vi "mapping final edition.vi"() -> ()   [LabVIEW 2018]
uses:
  <vilib>/DAQmx/read.llb/DAQmx Read (Analog 2D DBL NChan NSamp).vi
  <vilib>/DAQmx/create/channels.llb/DAQmx Create Channel (AI-Voltage-Basic).vi
  <vilib>/DAQmx/configure/timing.llb/DAQmx Timing (Sample Clock).vi
  <vilib>/DAQmx/miscellaneous.llb/DAQmx Fill In Error Info.vi
  <vilib>/Utility/file.llb/Write Delimited Spreadsheet (DBL).vi
panel:
  in  "Path":path
  out "array size":i32
  out "AI2":dbl=981483.9601007936 format="%.9f"
  out "AI2":sgl=0.9249536 format="%.3f"
  in  "Start Scan":bool
  in  "x start":sgl format="%.4f"
  out "sec":sgl=9.0 format="%.3f"
  out "min":sgl=2.0 format="%.3f"
  out "hr":sgl format="%.3f"
  out "scaled data":sgl[][](array[numeric])=[[0.08995186, -0.065358415, 0.046570934, -0.028403355, 0.011250414, 0.0097677205, -0.036845274, 0.08059889, -0.15414652, 3.8100245, 5.301704, 4.7763147, 5.1208405, 4.852381, 5.0800614, 4.8759155, 5.0671434, 4.879784, 5.073785, 4.854985, 5.1510253, 4.4088683, 0.19852792, -0.05369336, 0.042853996, -0.04278115, 0.046836343, -0.05056593, 0.057532918, -0.06434656, 0.07648512, -0.09306003, 0.12637737, -0.20857362, 0.7113754, 4.8934565, 4.9863224, 4.9517126, 5.008813, 4.9254646, 5.0359926, 4.8951178, 5.072542, 4.84753, 5.14237, 4.7289605, 5.41226, 3.039946, -0.3712578, 0.1811235, -0.102439806, 0.057444878, -0.02437124, -0.0019917544, 0.0284711, -0.055142883, 0.08947336, -0.13621256, 0.21908402, -0.42042786, 2.049878, 5.3894496, 4.758692, 5.1075525, 4.8870254, 5.0276275, 4.9465346, 4.976245, 4.9966516, 4.9206614, 5.0678873, 4.810496, 5.2940927, 1.5762044, -0.37725365, 0.20376839, -0.13209367, 0.091401376, -0.061783113, 0.038824435, -0.016206224, -0.005852878, 0.033383638, -0.07024288, 0.13338381, -0.2740278, 3.4729016, 5.3619275, 4.748465, 5.1354837, 4.846731, 5.0798483, 4.8825455, 5.0552025, 4.899335, 5.0453405, 4.898891, 5.074322, 4.648711, 0.41327354, -0.12288489, 0.0801944, -0.06521296, 0.05908707, -0.05554355, 0.055086855, -0.055220723, 0.0584478, -0.06400715, 0.07833402, -0.11937849, 0.401842, 4.63731, 5.0785136, 4.8963833, 5.0473413, 4.897698, 5.056591, 4.88092, 5.0812073, 4.844774, 5.1375537, 4.7452354, 5.367524, 3.4397311, -0.28283846, 0.13752055, -0.072798684, 0.035415, -0.007555047, -0.01475798, 0.03739533, -0.060410146, 0.09001565, -0.13058291, 0.20192842, -0.3742972, 1.560797, 5.291227, 4.811963, 5.0674405, 4.921157, 4.9965672, 4.9762244, 4.9467287, 5.0273952, 4.8875346, 5.1069274, 4.759733, 5.3872814, 2.030668, -0.41930884, 0.21865785, -0.13621894, 0.08957672, -0.05563924, 0.028855167, -0.002696095, -0.023640106, 0.056296494, -0.10112171, 0.17909977, -0.3670662, 3.0687323, 5.4088187, 4.730429, 5.1410356, 4.8483744, 5.071446, 4.8960123, 5.034976, 4.926784, 5.007408, 4.9539905, 4.9831657, 4.9024124, 0.72391576, -0.2121617, 0.12789325, -0.0943156, 0.07678369, -0.06477019, 0.057225406, -0.050254583, 0.045999296, -0.041641697, 0.040820073, -0.050278828, 0.18801892, 4.394757, 5.155556, 4.8520226, 5.076152, 4.877726, 5.069264, 4.873699, 5.082649, 4.849418, 5.124974, 4.770708, 5.312019, 3.7631257, -0.1722489, 0.08832625, -0.04115682, 0.012989575, 0.009221593, -0.026924489, 0.045944422, -0.065192536, 0.090805486, -0.1260621, 0.18888147, -0.34058186, 1.3266691, 5.213644, 4.8505197, 5.040275, 4.943368, 4.9778323, 4.993703, 4.9309473, 5.0431857, 4.8718643, 5.123718, 4.7399697, 5.416989, 2.3209786, -0.4270834, 0.2178795, -0.13206305, 0.08381564, -0.048057344, 0.020409431, 0.007566642, -0.03510993, 0.07040888, -0.11812037, 0.20245795, -0.40821925, 2.750202, 5.425666, 4.7273817, 5.137802, 4.8552256, 5.06122, 4.9094777, 5.01756, 4.9486656, 4.97851, 4.9933968, 4.920391, 5.0557537, 0.97315127, -0.27107772, 0.15618311], [1.6148105, 0.6412399, 0.12259479, 0.10007006, 0.05627404, 0.11792919, 0.07558805, 0.096587755, 0.13539684, 0.18154798, 0.14659481, 0.14001909, 0.15269747, 0.32605436, 1.2285366, 1.8071078, 1.723693, 1.8642299, 1.8861247, 1.7781298, 1.7665774, 1.6843293, 1.6618632, 1.8358308, 1.7840756, 1.886492, 1.4087651, 0.34988096, 0.17499523, 0.13713227, 0.14069235, 0.14307298, 0.15526807, 0.16397195, 0.16420785, 0.15337072, 0.103284605, 0.13004267, 0.0764462, 0.37955138, 1.4378004, 1.7283472, 1.6601341, 1.9107368, 1.981662, 1.9060649, 1.7642057, 1.8262956, 1.8092386, 1.8622408, 1.7110121, 1.835776, 1.0515572, 0.23552063, 0.18500735, 0.110096216, 0.11694353, 0.05356826, 0.11541723, 0.099398084, 0.09107675, 0.13544913, 0.09703531, 0.11242456, 0.118112795, 0.69184244, 1.4759477, 1.6194212, 1.8840069, 1.9284915, 1.8578812, 1.8474318, 1.8391486, 1.8397951, 1.8988006, 1.9207095, 1.7646545, 1.7554979, 0.7396219, 0.22156206, 0.15757602, 0.12271975, 0.1853172, 0.1761696, 0.16238572, 0.17065349, 0.12731779, 0.09591067, 0.09957277, 0.15292062, 0.100816004, 0.977814, 1.6875081, 1.8349446, 1.8618723, 1.7646685, 1.7791893, 1.7086927, 1.8239698, 1.9180751, 1.8788452, 1.7875822, 1.9220088, 1.4754479, 0.44321483, 0.13592602, 0.084151655, 0.08818737, 0.1107886, 0.15709913, 0.18759453, 0.15712845, 0.18021806, 0.17567357, 0.17235321, 0.12586543, 0.40349913, 1.447578, 1.674117, 1.8619998, 1.9170333, 1.8629906, 1.8370001, 1.8740305, 1.9876027, 1.8765373, 1.7414004, 1.6534603, 1.8096567, 1.1517842, 0.287448, 0.20285116, 0.066186704, 0.08846406, 0.11164929, 0.13587119, 0.15773286, 0.14254764, 0.10292374, 0.12034805, 0.15531144, 0.12162699, 0.6911105, 1.593376, 1.892207, 1.8803179, 1.9277658, 1.9091481, 1.860953, 1.9320847, 1.8267941, 1.8986298, 1.8120731, 1.6568379, 1.6279173, 0.781555, 0.19091108, 0.12488488, 0.08304486, 0.105652474, 0.11557407, 0.1490494, 0.09324315, 0.07362821, 0.0935173, 0.14308317, 0.15568249, 0.11385268, 0.87998796, 1.6663209, 1.8585353, 2.016943, 1.9768472, 1.8131237, 1.851382, 1.9297907, 1.8807145, 1.8564926, 1.8491366, 1.9471296, 1.5421423, 0.546228, 0.2057074, 0.20138735, 0.111848205, 0.08376657, 0.14174303, 0.16643672, 0.078453206, 0.116940975, 0.12531969, 0.098607525, -0.00568714, 0.2587199, 1.2634019, 1.6675119, 1.648064, 1.7753998, 1.9649504, 1.7998588, 1.7356408, 1.7368636, 1.6777064, 1.8816746, 1.8367412, 1.8527502, 1.2181253, 0.3530853, 0.21028247, 0.09459221, 0.1144762, 0.10214721, 0.092193745, 0.062590905, 0.115664594, 0.09098494, 0.115862235, 0.09943251, 0.069180645, 0.4846417, 1.4973682, 1.8450817, 1.8296045, 1.8144448, 1.7862815, 1.799637, 1.9097167, 1.8960272, 1.7957402, 1.7565843, 1.7647425, 1.8072952, 0.8449825, 0.1833395, 0.18335354, 0.031213127, 0.09104742, 0.12451765, 0.15377748, 0.09247936, 0.13039716, 0.17976157, 0.1752885, 0.16731273, 0.18515654, 0.9803604, 1.7406315, 1.85674, 1.8916562, 1.7167296, 1.7266883, 1.7743402, 1.8966228, 1.7989038, 1.7762464, 1.8464664], [-1.4767952, -0.52093244, -0.065139994, -0.04381245, -0.015159501, -0.023012077, 0.030354373, 0.004124446, -0.037436225, -0.03062673, -0.049429834, -0.038981438, -0.05951384, -0.12666832, -0.96224815, -1.4578644, -1.417214, -1.6564966, -1.5031904, -1.4855494, -1.5529104, -1.5899595, -1.6205446, -1.4851049, -1.3304464, -1.4843547, -1.1244048, -0.3124867, -0.09511276, -0.0067108776, 0.008348133, -0.06884276, -0.028149867, 0.0060778856, 0.014657993, 0.0035960134, 0.029784627, -0.001404034, -0.010573929, -0.23944686, -1.1427158, -1.592673, -1.6138891, -1.5006585, -1.5761764, -1.6237564, -1.6302592, -1.4553976, -1.4390112, -1.5583963, -1.6095014, -1.6356761, -0.8941107, -0.14872715, -0.04852324, -0.016287742, -0.0072004925, 0.05171574, 0.024102116, -0.03878735, -0.029223012, 0.0013796147, 0.0007109344, -0.09832217, -0.026550805, -0.57925135, -1.3799185, -1.4696552, -1.5014336, -1.6099834, -1.6062907, -1.5134172, -1.4725603, -1.4464005, -1.471114, -1.6949456, -1.6740988, -1.443826, -0.5317577, -0.096025616, -0.095088966, -0.01003298, -0.030934773, -0.03786698, -0.066740304, -0.028596912, -0.0075047743, -0.045842268, -0.028847354, 0.017677061, -0.06430727, -0.91461426, -1.5800095, -1.6365865, -1.669164, -1.6613489, -1.5563904, -1.6387641, -1.621947, -1.6419398, -1.5808084, -1.4260033, -1.746947, -1.4109493, -0.31155756, -0.03549656, -0.0893977, -0.0493835, -0.02766151, -0.055632003, -0.020448817, -0.03490928, -0.0065092742, -0.0044493936, -0.008321209, 0.03713632, -0.22255462, -1.256689, -1.6435188, -1.58099, -1.6661974, -1.6825287, -1.7567831, -1.6967863, -1.6964307, -1.5608094, -1.5687697, -1.5021436, -1.7775272, -1.1238, -0.18753046, -0.06339442, 0.033160567, -0.037432462, -0.0655407, 0.012275046, 0.019751964, -0.074713096, -0.059357315, 0.017791009, -0.004530791, 0.051316284, -0.45699736, -1.4750546, -1.6812614, -1.6400126, -1.5128337, -1.5886396, -1.4835271, -1.558737, -1.5912981, -1.5443467, -1.5120009, -1.5561036, -1.5510322, -0.6751001, -0.13700025, -0.070947714, 0.029946156, -0.06867997, -0.0646341, -0.023216186, 0.022019707, -0.00063267536, -0.049820524, 0.08989921, 0.031814445, -0.01631529, -0.76614785, -1.5538985, -1.7605923, -1.8131211, -1.615681, -1.6916823, -1.5543268, -1.4462615, -1.5637659, -1.6425695, -1.5686895, -1.6034069, -1.3314981, -0.39967144, -0.1255188, -0.042046838, -0.05730996, -0.059426185, -0.054224525, -0.0747444, 0.004988471, -0.03528243, -0.036589727, -0.0626456, -0.030736923, -0.1435518, -1.0285323, -1.4818504, -1.4843473, -1.4634567, -1.4524511, -1.5054933, -1.5445257, -1.5867013, -1.5180717, -1.6029373, -1.6105895, -1.7413071, -1.0346706, -0.19276091, -0.12739836, -0.015712976, -0.051736392, -0.0066845864, 0.0036811642, -0.018952433, -0.008254843, 0.023332015, 0.015603406, 0.005991487, 0.005503129, -0.3153793, -1.1979393, -1.4788326, -1.5864795, -1.5806519, -1.5993572, -1.5863644, -1.4998145, -1.6164098, -1.6253455, -1.5748917, -1.7109123, -1.6193199, -0.67024153, -0.121727124, -0.092952706, -0.02475514, -0.026037404, 0.034906138, -0.02021716, -0.03959001, -0.008375058, -0.047745623, -0.024242997, -0.06765317, -0.029479712, -0.7310273, -1.4417034, -1.4696852, -1.4992273, -1.62077, -1.7575307, -1.5015112, -1.5808134, -1.6111705, -1.6930485, -1.6120521]] format="%0.6f"
  in  "Physical Channel":tag="Dev2/ai0:2"
  in  "AI Rate":dbl=5120.0 format="%.2f"
  out "X Position":sgl=5.7001514 format="%.4f"
  out "AI0":dbl=1080521.7918445107 format="%.9f"
  out "AI1":dbl=981483.9601007936 format="%.9f"
  out "Y Position":sgl=0.6143307 format="%.4f"
  out "necessary time (s)":dbl=129.0
  in  "Time/Step(ms)":u32=1000 min=1 step=1
  out "For_Home":dbl=0.5
  in  "Motor HWSerialNum A":u32=83827753
  out "error":errorcluster
  in  "Channel A":i32
  in  "Channel B":i32
  in  "Both Channels":i32=10
  in  "MG17Motor A":refnum<k7>(container)
  in  "MG17Motor B":refnum<k7>(container)
  in  "Motor HWSerialNum B":u32=83827752
  in  "Error":errorcluster
  in  "Z Scale.Range:Minimum":dbl=0.5
  in  "Z Scale.Range:Maximum":dbl=10.0
  in  "Pixels(Y)":i32=10
  out "x .and. y?":bool=TRUE
  out "AI1 Reading":sgl=1916.9768 caption="AI1" format="%.3f"
  out "AI0 Reading":sgl=1773.1146 caption="AI0" format="%.3f"
  out "AI2":dbl[][](graph)
  out "Outphase Array":dbl[][](array[numeric])=[[2562.4082924284185, 1817.6676888834427, 2051.3325671838757, 1598.5840726397216, 2356.139803338449, 2083.283068035537, 2141.9285945761453, 2438.1745524803077, 1984.8193530672331, 2518.2976810936884], [2013.6293646842878, 2905.788176064875, 2403.5143450391743, 2075.1285214946324, 1794.2852932607746, 2154.2324476248573, 2573.051600709472, 2289.9591852377134, 1840.6423205131646, 3056.691954941658], [1462.7563247041599, 2489.6853377240786, 3113.7141928608366, 2094.263243597831, 1980.880488063484, 2798.2521113290636, 3180.218346584931, 1955.014012814602, 1954.9062009375507, 2330.0172899718864], [2654.506466159619, 1706.9104786367188, 2763.849371509579, 2665.4676788285865, 3132.939147321313, 1990.492248608471, 3191.66238810395, 2902.203788288949, 2369.1083072617203, 2413.0030199350244], [2875.5255335084453, 1413.9419064107196, 2133.996309941279, 1582.8516778375904, 2285.5732989580556, 2032.7550230687993, 1403.1269673599186, 2348.5457130522527, 2793.543648369003, 2638.42704917987], [2508.860871301475, 2017.0923640774959, 2103.4938570285726, 2506.6668144539026, 2520.3189193813937, 1623.1935507015144, 2117.008235660878, 1990.9220243912062, 2369.004550581991, 1817.1745751417288], [2127.008781202753, 1894.076946993543, 2350.908791062092, 1608.5249433544752, 2367.4088747592477, 2261.8591956234536, 2856.9839458223373, 1944.1817298861051, 2606.7766866868633, 1847.702813397054], [1332.3239444506978, 3089.345384527674, 3117.6849510516045, 1823.2018060552239, 2907.347843840017, 2513.6901896156223, 1883.004697534108, 2598.892861462688, 2158.04090585742, 2821.9623698891833], [2783.620807424688, 3090.3816841375274, 2126.982362670075, 1802.3502961996567, 2121.8058461401215, 1389.8670829981122, 2695.1174997292997, 1862.877057878669, 1123.7561431306951, 3173.8482288755017], [3289.294215227313, 3427.646935048104, 1868.9893279501098, 1265.6961355991489, 3028.863630242435, 2568.628200265615, 2625.960251038055, 2112.3260575013605, 2293.5876318191563, 1916.9768566871817], [0.0, 0.0, 0.0, 0.0, 0.0, 0.0, 0.0, 0.0, 0.0, 0.0], [0.0, 0.0, 0.0, 0.0, 0.0, 0.0, 0.0, 0.0, 0.0, 0.0], [0.0, 0.0, 0.0, 0.0, 0.0, 0.0, 0.0, 0.0, 0.0, 0.0], [0.0, 0.0, 0.0, 0.0, 0.0, 0.0, 0.0, 0.0, 0.0, 0.0], [0.0, 0.0, 0.0, 0.0, 0.0, 0.0, 0.0, 0.0, 0.0, 0.0], [0.0, 0.0, 0.0, 0.0, 0.0, 0.0, 0.0, 0.0, 0.0, 0.0], [0.0, 0.0, 0.0, 0.0, 0.0, 0.0, 0.0, 0.0, 0.0, 0.0], [0.0, 0.0, 0.0, 0.0, 0.0, 0.0, 0.0, 0.0, 0.0, 0.0], [0.0, 0.0, 0.0, 0.0, 0.0, 0.0, 0.0, 0.0, 0.0, 0.0], [0.0, 0.0, 0.0, 0.0, 0.0, 0.0, 0.0, 0.0, 0.0, 0.0]]
  out "Inphase Array":dbl[][](array[numeric])=[[2044.6463625125714, 2048.007662191087, 1857.2525864253337, 2367.536167113699, 1677.5847421288915, 3518.7700021734063, 3017.990323192611, 1790.35736608951, 973.9359143332003, 1961.5367899300145], [1674.8440274838545, 2393.3161888851737, 3047.069407355723, 2831.9502902122717, 2575.6596526949597, 2640.3955094250277, 2707.38612778617, 2752.6705551580535, 2601.6534846507584, 2428.802308846195], [2310.539174707911, 2019.4980579908167, 1695.4316967259595, 3165.8313269644823, 2974.8805843760015, 2521.9709412910042, 1332.5610352925755, 1952.563600677248, 2877.336113219085, 1895.061160929894], [3252.8926277691635, 2822.4440682237696, 2634.978174426852, 2361.470345238801, 2106.861238475591, 2470.3862405323457, 2504.170845974706, 2514.8891074351964, 1680.5844638621936, 2858.877309939785], [2768.0539491905397, 2186.0164703118107, 2539.6366460966865, 2640.577817303329, 3117.019873675447, 2573.625813695958, 1976.3462073162439, 2035.7740034242272, 1545.9525168596529, 2242.6229061407557], [1874.3233177350737, 2505.741725715464, 2783.8180046186562, 1842.768823260741, 2555.264741602122, 2882.3282081275916, 2818.5003810212797, 3251.099795547098, 2569.4618761698066, 1322.899149168236], [1540.9844582418293, 2057.077993816449, 2495.5409296646358, 1977.5648561441858, 2223.188598020489, 2486.5520399883585, 1586.5726572114816, 2615.9088005342264, 1254.4943744059751, 2253.562060012856], [2955.7185549552687, 2750.74135698765, 1818.3861337580702, 2572.2228754086773, 2137.553351193629, 1375.2105871652152, 3355.1487666885364, 2141.5017884888475, 2734.5506302466356, 1843.7281765812454], [1858.2546438169445, 1583.66230481497, 2611.782079607164, 3046.8759742374796, 1529.7603908309666, 1274.6513951532384, 2276.057074441497, 2421.2195908700114, 2331.4669215367194, 3086.2871139714543], [2460.676783449499, 1393.87787290715, 2469.907081701711, 2303.007218218374, 1704.4213840891673, 1594.5417502298358, 2147.1556828119224, 2407.7757693353487, 1540.0436035810508, 1773.1145717006036], [0.0, 0.0, 0.0, 0.0, 0.0, 0.0, 0.0, 0.0, 0.0, 0.0], [0.0, 0.0, 0.0, 0.0, 0.0, 0.0, 0.0, 0.0, 0.0, 0.0], [0.0, 0.0, 0.0, 0.0, 0.0, 0.0, 0.0, 0.0, 0.0, 0.0], [0.0, 0.0, 0.0, 0.0, 0.0, 0.0, 0.0, 0.0, 0.0, 0.0], [0.0, 0.0, 0.0, 0.0, 0.0, 0.0, 0.0, 0.0, 0.0, 0.0], [0.0, 0.0, 0.0, 0.0, 0.0, 0.0, 0.0, 0.0, 0.0, 0.0], [0.0, 0.0, 0.0, 0.0, 0.0, 0.0, 0.0, 0.0, 0.0, 0.0], [0.0, 0.0, 0.0, 0.0, 0.0, 0.0, 0.0, 0.0, 0.0, 0.0], [0.0, 0.0, 0.0, 0.0, 0.0, 0.0, 0.0, 0.0, 0.0, 0.0], [0.0, 0.0, 0.0, 0.0, 0.0, 0.0, 0.0, 0.0, 0.0, 0.0]]
  out "Ratio Array":dbl[][](array[numeric])=[[0.7979393325233274, 1.1267228188718796, 0.9053883393344746, 1.4810207405633764, 0.7120056032973499, 1.689050353340357, 1.4090060382194136, 0.7343023756310696, 0.4906924717496996, 0.7789137895239316], [0.831753875294945, 0.8236375275386695, 1.267755864925391, 1.364710793032005, 1.4354794426332196, 1.2256780888878487, 1.0522082522712166, 1.2020609681182188, 1.4134486943261342, 0.7945852394185899], [1.5795790014274689, 0.8111459016089644, 0.544504598595872, 1.5116682855617305, 1.5017971060355364, 0.9012665195821701, 0.4190155800854185, 0.9987466012410693, 1.4718537962788942, 0.8133249350062803], [1.2254227553173958, 1.65353959891207, 0.9533725685592123, 0.8859497205670919, 0.6724871245191512, 1.241093122698349, 0.7845976614908642, 0.8665446298372791, 0.7093742648704224, 1.184779830908279], [0.9626254112281246, 1.546044049193645, 1.1900848348545503, 1.668240842951722, 1.3637803150292447, 1.266077704636843, 1.4085298431936473, 0.8668232396372918, 0.5534019551698252, 0.8499848069848487], [0.7470814102030161, 1.2422543312048324, 1.3234257829262785, 0.7351470935965628, 1.0138656350003934, 1.775714428437633, 1.3313601400050354, 1.632961891885864, 1.084616690811577, 0.7279978309541656], [0.7244842954388057, 1.0860583024790185, 1.0615217992090633, 1.2294275350310089, 0.9390809596616785, 1.09933989029895, 0.5553313169755358, 1.3455063178108728, 0.4812435145721672, 1.2196561285034893], [2.218468389212864, 0.8903961890321975, 0.5832488408248958, 1.4108272967182252, 0.7352244953154125, 0.5470883376346007, 1.7818058399335261, 0.8240054140914392, 1.2671449474495295, 0.6533496676830767], [0.6675674498697756, 0.5124487738662427, 1.2279284141916924, 1.690501552701473, 0.7209709567036149, 0.9171030890260818, 0.8445112595907625, 1.299720548186443, 2.07470894445252, 0.9724116880865881], [0.7480865567020885, 0.4066573656272997, 1.321520163205363, 1.8195577543801127, 0.5627263529037597, 0.6207756148067473, 0.8176649596897521, 1.1398693685497927, 0.6714561860274626, 0.9249535619145693], [0.0, 0.0, 0.0, 0.0, 0.0, 0.0, 0.0, 0.0, 0.0, 0.0], [0.0, 0.0, 0.0, 0.0, 0.0, 0.0, 0.0, 0.0, 0.0, 0.0], [0.0, 0.0, 0.0, 0.0, 0.0, 0.0, 0.0, 0.0, 0.0, 0.0], [0.0, 0.0, 0.0, 0.0, 0.0, 0.0, 0.0, 0.0, 0.0, 0.0], [0.0, 0.0, 0.0, 0.0, 0.0, 0.0, 0.0, 0.0, 0.0, 0.0], [0.0, 0.0, 0.0, 0.0, 0.0, 0.0, 0.0, 0.0, 0.0, 0.0], [0.0, 0.0, 0.0, 0.0, 0.0, 0.0, 0.0, 0.0, 0.0, 0.0], [0.0, 0.0, 0.0, 0.0, 0.0, 0.0, 0.0, 0.0, 0.0, 0.0], [0.0, 0.0, 0.0, 0.0, 0.0, 0.0, 0.0, 0.0, 0.0, 0.0], [0.0, 0.0, 0.0, 0.0, 0.0, 0.0, 0.0, 0.0, 0.0, 0.0]]
  in  "st(mm/step)":dbl=2.0 format="%_1f"
  in  "Pixels(X)":i32=10
  # "Necessary Time"
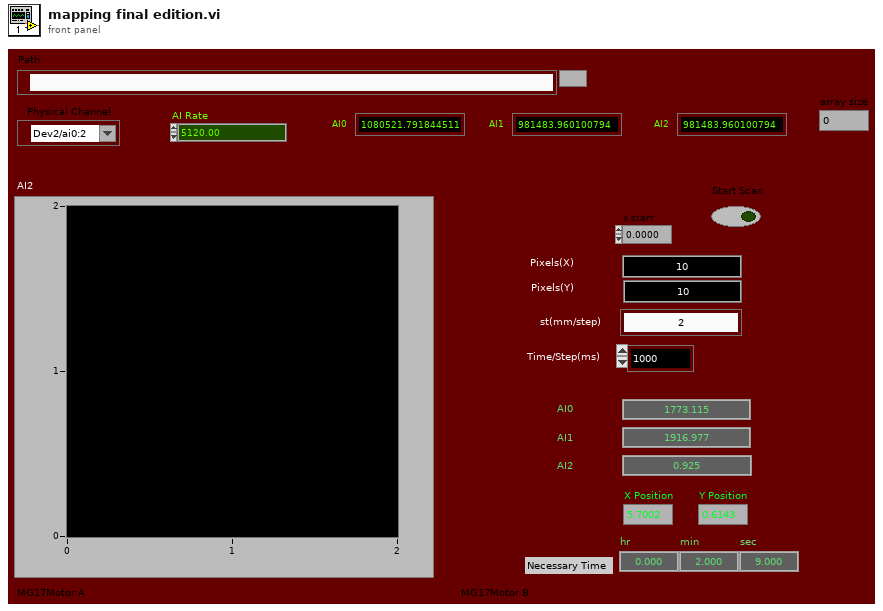
[diagram p1: front panel]
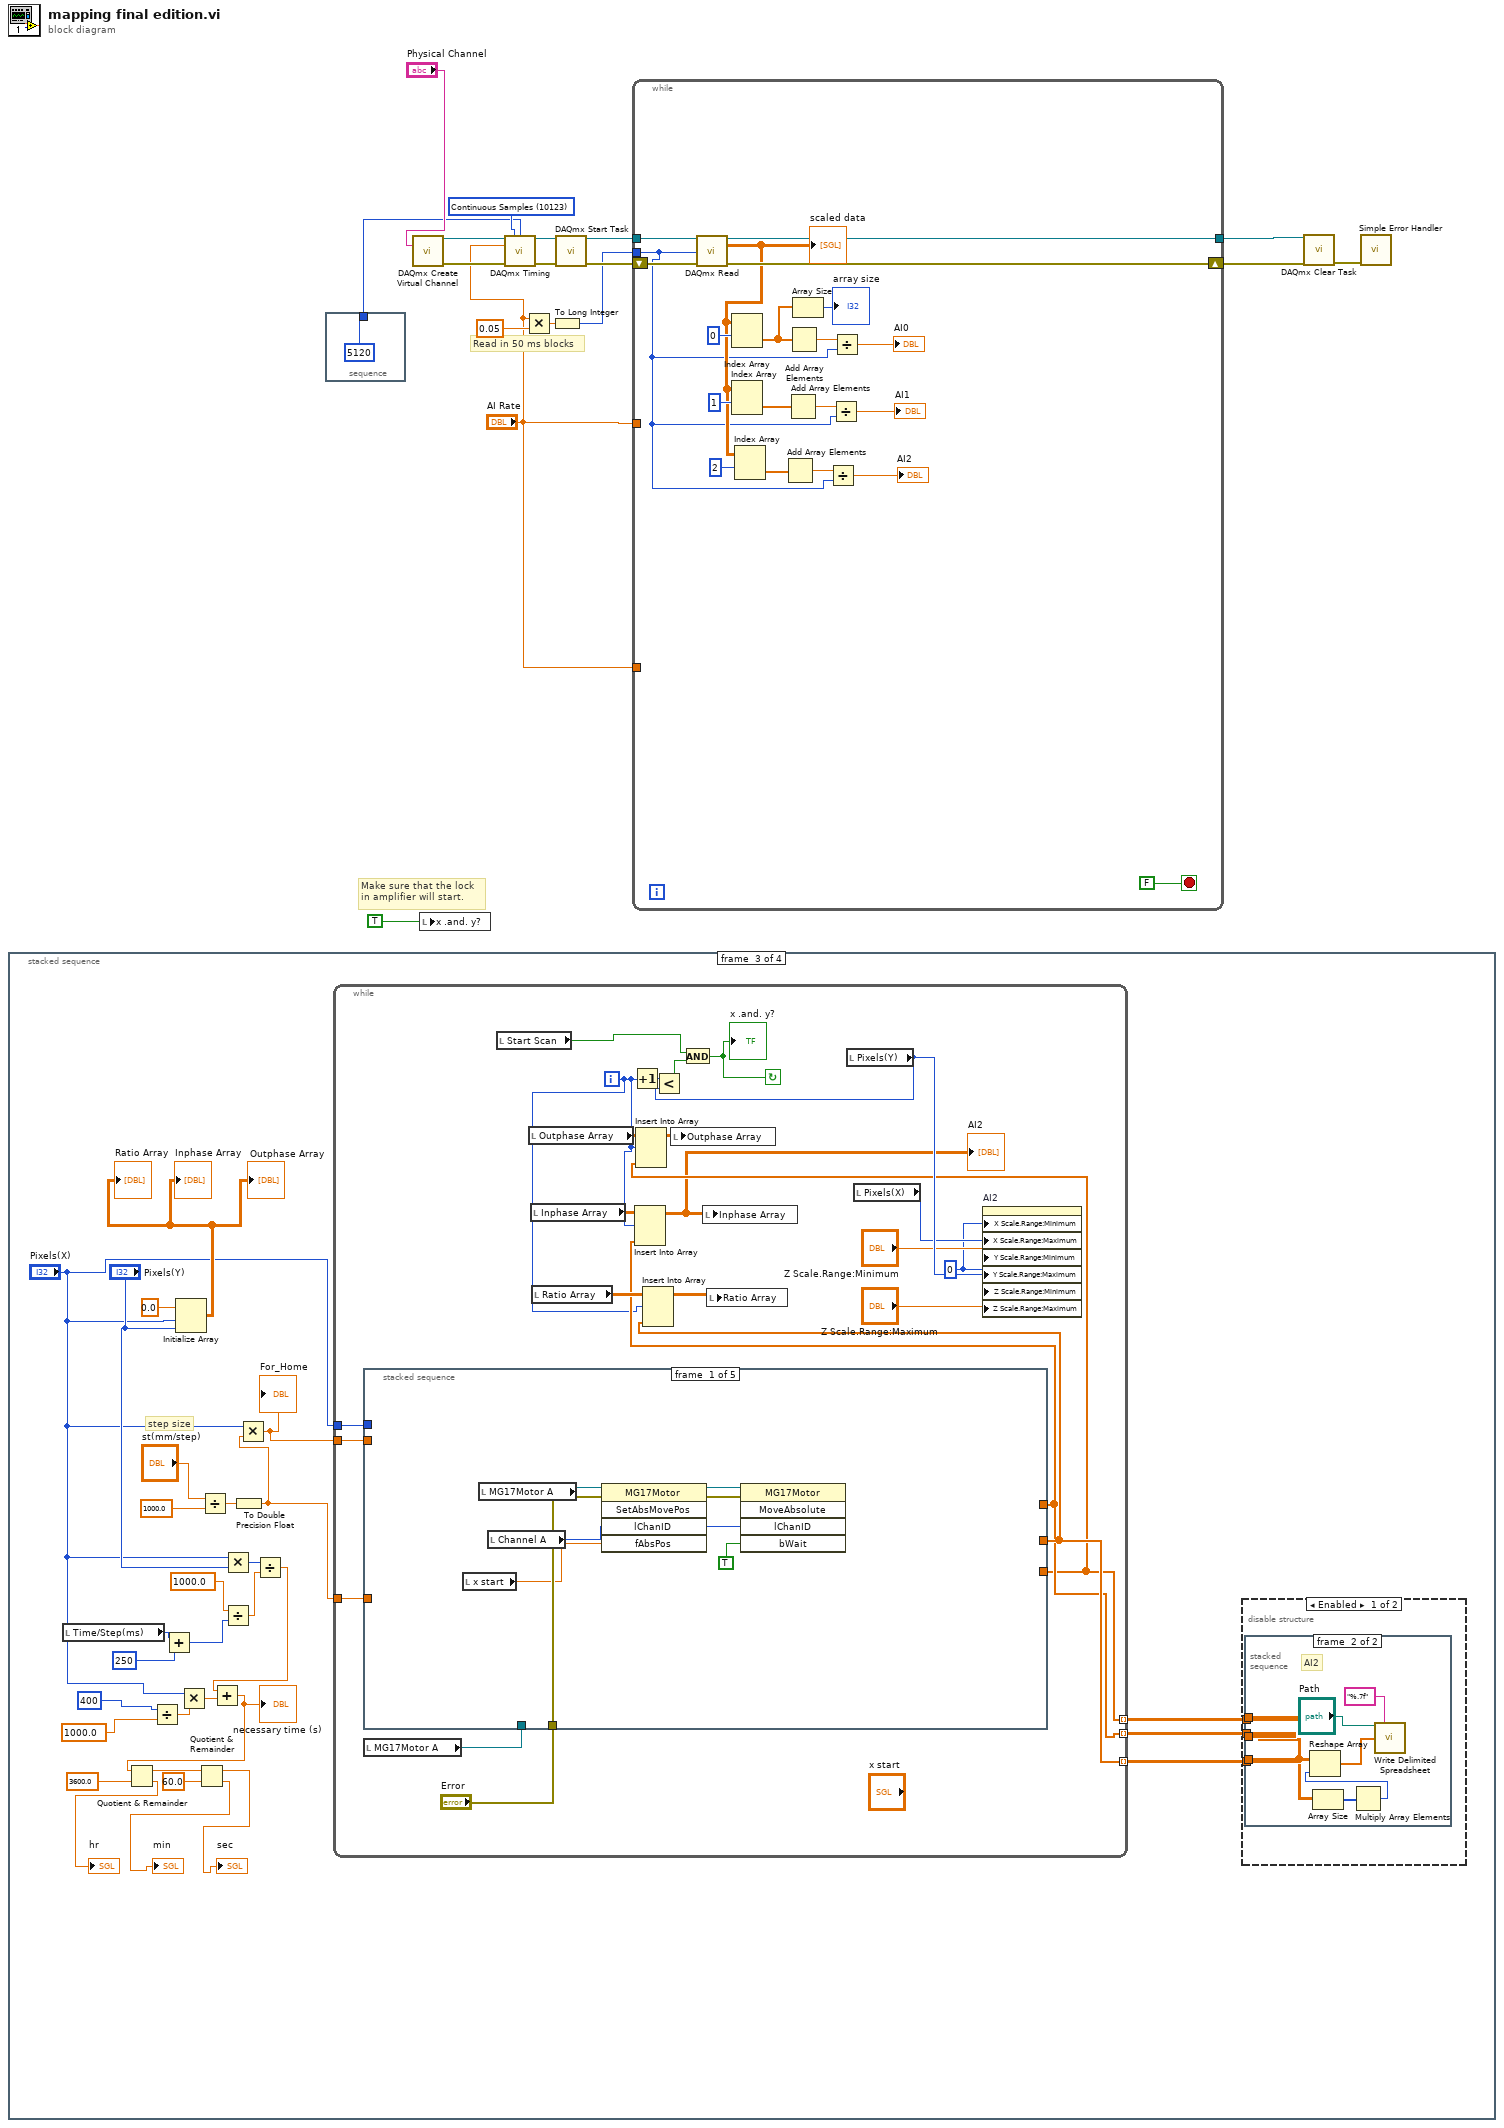
[diagram p0: block diagram]
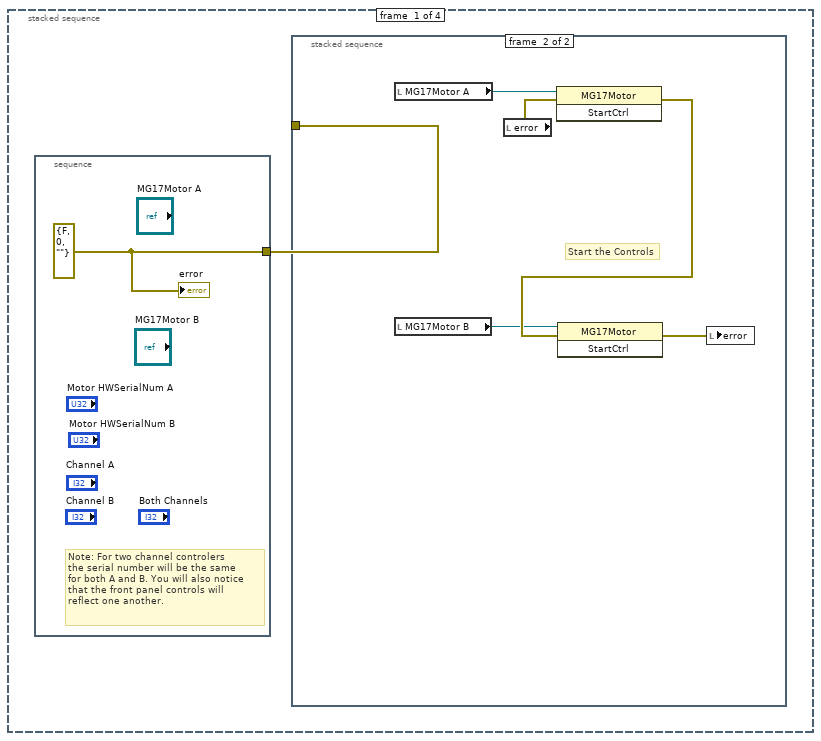
[diagram p2: hidden frame]
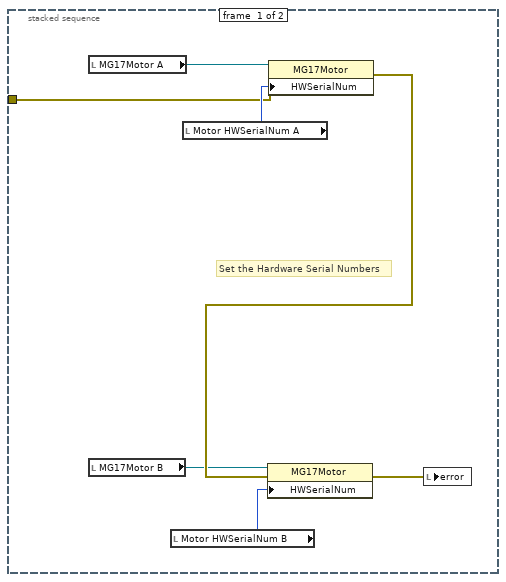
[diagram p3: hidden frame]
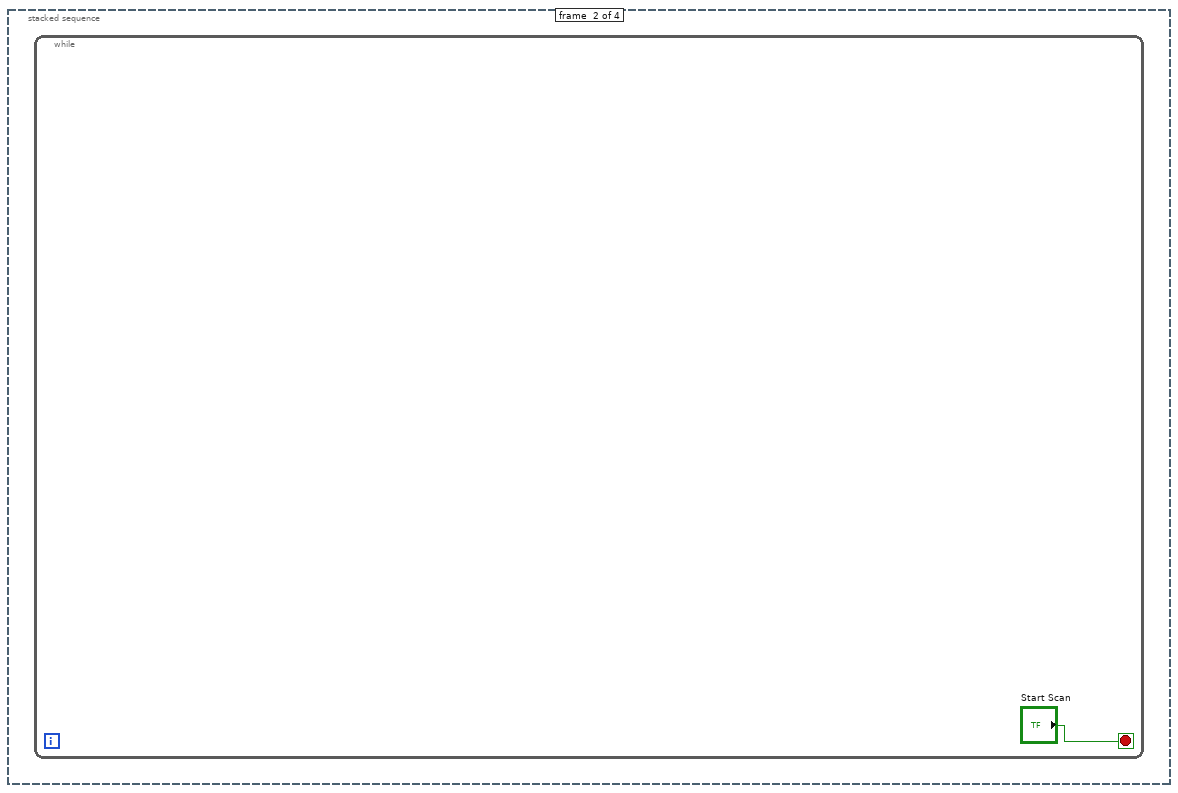
[diagram p4: hidden frame]
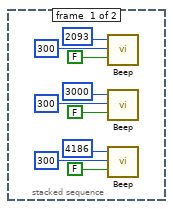
[diagram p5: hidden frame]
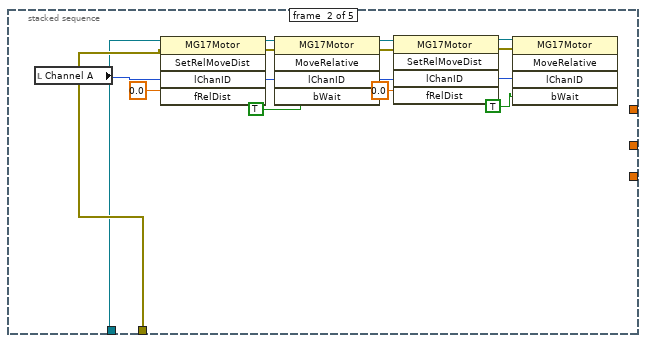
[diagram p7: hidden frame]
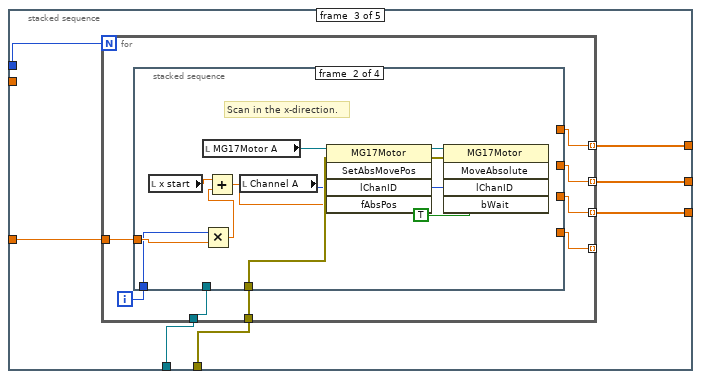
[diagram p8: hidden frame]
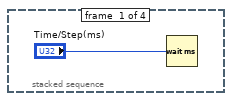
[diagram p9: hidden frame]
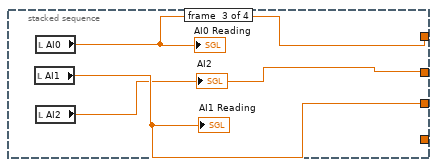
[diagram p10: hidden frame]
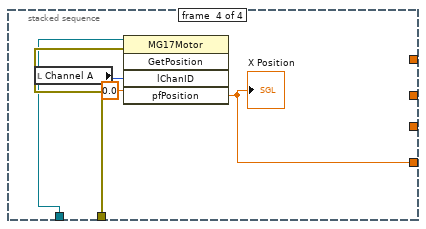
[diagram p11: hidden frame]
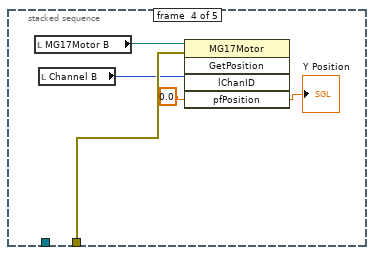
[diagram p12: hidden frame]
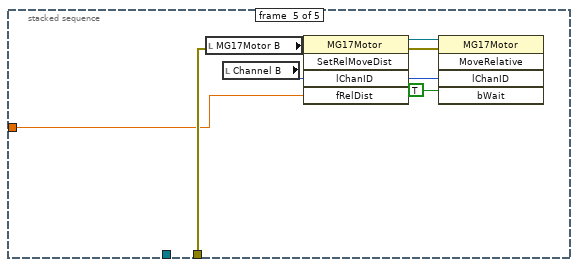
[diagram p13: hidden frame]
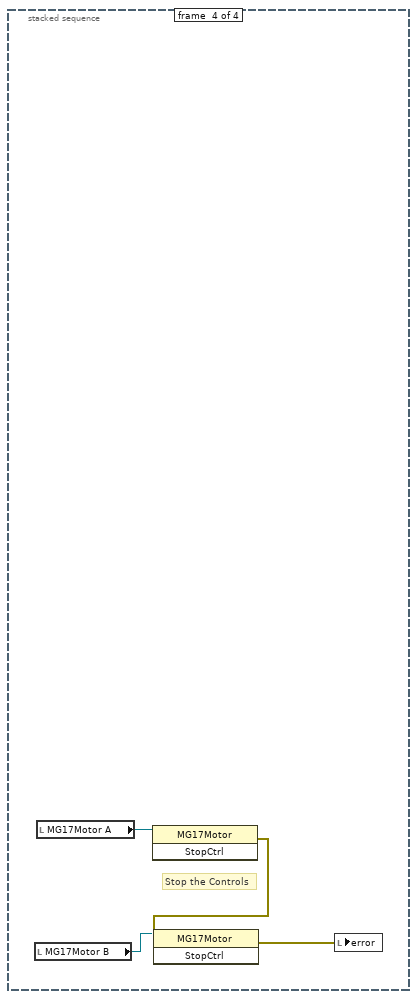
[diagram p14: hidden frame]
diagram:
  w2 = 10123 items=["Finite Samples"=10178, "Continuous Samples"=10123, "Hardware Timed Single Point"=12522] ("sample mode")
  # "Read in 50 ms blocks"
  # "Make sure that the lock in amplifier will start."
  n1 = stacked-sequence {
    frame #0 {
      n2 = stacked-sequence {
        tunnel: [w19] -> w18
        frame #0 {
          w19 = errorcluster {"status"=FALSE, "code"=0, "source"=""} ("error in (no error)")
          # "Note: For two channel controlers\nthe serial number will be the same\nfor both A and B. You will also notice\nthat the front panel controls will\nreflect one another."
          "error" <- w19
        }
      }
      n3 = stacked-sequence {
        tunnel: w18 -> [w20 _]
        frame #0 {
          # "Set the Hardware Serial Numbers"
          n4 = local read "MG17Motor A"() -> (w25:refnum<k7>)
          n5 = local read "MG17Motor B"() -> (w22:refnum<k7>)
          n6 = local read "Motor HWSerialNum B"() -> (w21:u32)
          n7 = local read "Motor HWSerialNum A"() -> (w26:u32)
          n8 = property class="MG17Motor"(reference=w25, error in=w20, "HWSerialNum"=w26) -> (error out=w24:errorcluster)  [unwired: 1 out]
          n9 = property class="MG17Motor"(reference=w22, error in=w24, "HWSerialNum"=w21) -> (error out=w23:errorcluster)  [unwired: 1 out]
          n10 = local write "error"(w23) -> ()
        }
        frame #1 {
          # "Start the Controls"
          n11 = local read "MG17Motor A"() -> (w31:refnum<k7>)
          n12 = local read "MG17Motor B"() -> (w27:refnum<k7>)
          n13 = local read "error"() -> (w30:errorcluster)
          n14 = invoke class="MG17Motor" method="StartCtrl"(reference=w31, error in=w30) -> (error out=w28:errorcluster)  [unwired: 1 in, 2 out]
          n15 = invoke class="MG17Motor" method="StartCtrl"(reference=w27, error in=w28) -> (error out=w29:errorcluster)  [unwired: 1 in, 2 out]
          n16 = local write "error"(w29) -> ()
        }
      }
    }
    frame #1 {
      n17 = while {
        stop <- "Start Scan" stop-if-true
      }
    }
    frame #2 {
      # "step size"
      n18 = local read "Time/Step(ms)"() -> (w45:u32)
      n19 = Divide(x=u32 400 ("y"), y=1000.0) -> (x/y=w54:dbl)
      n20 = Add(x=w45, y=u32 250) -> (x+y=w41:u32)
      n21 = Initialize Array(0.0, "Pixels(X)", "Pixels(Y)") -> (→"Ratio Array" →"Inphase Array" →"Outphase Array":dbl[][])
      n22 = Multiply(x="Pixels(X)", y=w54) -> (x*y=w49:dbl)
      n23 = Divide(x="st(mm/step)", y=1000.0) -> (x/y=w59:dbl)
      n24 = Multiply(x="Pixels(X)", y="Pixels(Y)") -> (x*y=w46:i32)
      n25 = Divide(x=1000.0, y=w41) -> (x/y=w53:dbl)
      n26 = To Double Precision Float(number=w59) -> (double precision float=w34:dbl)
      n27 = Multiply(x="Pixels(X)", y=w34) -> (x*y=w33:dbl)
      "For_Home" <- w33
      n28 = Divide(x=w46, y=w53) -> (x/y=w48:dbl)
      n29 = Add(x=w48, y=w49) -> (x+y=w39:dbl)
      "necessary time (s)" <- w39
      n30 = Quotient & Remainder(x=w39, y=3600.0) -> (x-y*floor(x/y)=w43:dbl, floor(x/y)=→"hr":dbl)
      n31 = Quotient & Remainder(x=w43, y=60.0) -> (x-y*floor(x/y)=→"sec":dbl, floor(x/y)=→"min":dbl)
      n32 = while {
        tunnel: [w103] -> w55 mode=indexing
        tunnel: w34 -> [w93]
        tunnel: [w101] -> w57 mode=indexing
        tunnel: "Pixels(X)" -> [w98]
        tunnel: [w84] -> w56 mode=indexing
        tunnel: w33 -> [w88]
        i -> [w85]
        stop <- w90 continue-if-true
        w89 = 0
        n33 = local read "MG17Motor A"() -> (w87:refnum<k7>)
        n34 = stacked-sequence {
          tunnel: [_ _ w135 _ _] -> w103
          tunnel: [_ _ w134 _ _] -> w101
          tunnel: w98 -> [_ _ w129 _ _]
          tunnel: [_ _ w133 _ _] -> w84
          tunnel: "Error" -> [w112 w114 w132 w166 w177]
          tunnel: w93 -> [_ _ w131 _ w170]
          tunnel: w87 -> [_ w113 w130 _ _]
          tunnel: w88 -> [_ _ _ _ _]
          frame #0 {
            n35 = local read "x start"() -> (w109:sgl)
            n36 = local read "MG17Motor A"() -> (w111:refnum<k7>)
            n37 = local read "Channel A"() -> (w110:i32)
            n38 = invoke class="MG17Motor" method="SetAbsMovePos"(reference=w111, error in=w112, "lChanID"=w110, "fAbsPos"=w109) -> (reference out=w107:refnum<k7>, error out=w108:errorcluster, "lChanID"=w106:i32)  [unwired: 1 in, 2 out]
            n39 = invoke class="MG17Motor" method="MoveAbsolute"(reference=w107, error in=w108, "lChanID"=w106, "bWait"=TRUE) -> ()  [unwired: 1 in, 5 out]
          }
          frame #1 {
            n40 = local read "Channel A"() -> (w115:i32)
            n41 = invoke class="MG17Motor" method="SetRelMoveDist"(reference=w113, error in=w114, "lChanID"=w115, "fRelDist"=sgl 0.0) -> (reference out=w127:refnum<k7>, error out=w126:errorcluster, "lChanID"=w128:i32)  [unwired: 1 in, 2 out]
            n42 = invoke class="MG17Motor" method="MoveRelative"(reference=w127, error in=w126, "lChanID"=w128, "bWait"=TRUE) -> (reference out=w121:refnum<k7>, error out=w120:errorcluster, "lChanID"=w119:i32)  [unwired: 1 in, 2 out]
            n43 = invoke class="MG17Motor" method="SetRelMoveDist"(reference=w121, error in=w120, "lChanID"=w119, "fRelDist"=sgl 0.0) -> (reference out=w123:refnum<k7>, error out=w122:errorcluster, "lChanID"=w124:i32)  [unwired: 1 in, 2 out]
            n44 = invoke class="MG17Motor" method="MoveRelative"(reference=w123, error in=w122, "lChanID"=w124, "bWait"=TRUE) -> ()  [unwired: 1 in, 5 out]
          }
          frame #2 {
            n45 = for {
              N: w129 -> [_]
              tunnel: [w143] -> w135 mode=indexing
              tunnel: [w142] -> w133 mode=indexing
              tunnel: [w141] -> w134 mode=indexing
              tunnel: w131 -> [w140]
              tunnel: w132 -> [w139]
              tunnel: w130 -> [w138]
              tunnel: [w136] -> _ mode=indexing
              i -> [w137]
              n46 = stacked-sequence {
                tunnel: w140 -> [_ w155 _ _]
                tunnel: [_ _ w157 _] -> w143
                tunnel: [_ _ w158 _] -> w142
                tunnel: [_ _ w159 _] -> w141
                tunnel: w139 -> [_ w156 _ w162]
                tunnel: w138 -> [_ _ _ w161]
                tunnel: w137 -> [_ w154 _ _]
                tunnel: [_ _ _ w160] -> w136
                frame #0 {
                  n47 = Wait (ms)(milliseconds to wait="Time/Step(ms)") -> ()  [unwired: 1 out]
                }
                frame #1 {
                  # "Scan in the x-direction."
                  n48 = local read "x start"() -> (w152:sgl)
                  n49 = local read "MG17Motor A"() -> (w147:refnum<k7>)
                  n50 = Multiply(x=w154, y=w155) -> (x*y=w153:dbl)
                  n51 = Add(x=w152, y=w153) -> (x+y=w151:dbl)
                  n52 = local read "Channel A"() -> (w146:i32)
                  n53 = invoke class="MG17Motor" method="SetAbsMovePos"(reference=w147, error in=w156, "lChanID"=w146, "fAbsPos"=w151) -> (reference out=w150:refnum<k7>, error out=w149:errorcluster, "lChanID"=w148:i32)  [unwired: 1 in, 2 out]
                  n54 = invoke class="MG17Motor" method="MoveAbsolute"(reference=w150, error in=w149, "lChanID"=w148, "bWait"=TRUE) -> ()  [unwired: 1 in, 5 out]
                }
                frame #2 {
                  n55 = local read "AI1"() -> (w158:dbl)
                  "AI1 Reading" <- w158
                  n56 = local read "AI0"() -> (w159:dbl)
                  "AI0 Reading" <- w159
                  n57 = local read "AI2"() -> (w157:dbl)
                  "AI2" <- w157
                }
                frame #3 {
                  n58 = local read "Channel A"() -> (w163:i32)
                  n59 = invoke class="MG17Motor" method="GetPosition"(reference=w161, error in=w162, "lChanID"=w163, "pfPosition"=sgl 0.0) -> ("pfPosition"=w160:sgl)  [unwired: 1 in, 4 out]
                  "X Position" <- w160
                }
              }
            }
          }
          frame #3 {
            n60 = local read "MG17Motor B"() -> (w167:refnum<k7>)
            n61 = local read "Channel B"() -> (w165:i32)
            n62 = invoke class="MG17Motor" method="GetPosition"(reference=w167, error in=w166, "lChanID"=w165, "pfPosition"=sgl 0.0 ("pfCalibPosition")) -> ("pfPosition"=→"Y Position":sgl)  [unwired: 1 in, 4 out]
          }
          frame #4 {
            n63 = local read "MG17Motor B"() -> (w176:refnum<k7>)
            n64 = local read "Channel B"() -> (w175:i32)
            n65 = invoke class="MG17Motor" method="SetRelMoveDist"(reference=w176, error in=w177, "lChanID"=w175, "fRelDist"=w170) -> (reference out=w174:refnum<k7>, error out=w173:errorcluster, "lChanID"=w172:i32)  [unwired: 1 in, 2 out]
            n66 = invoke class="MG17Motor" method="MoveRelative"(reference=w174, error in=w173, "lChanID"=w172, "bWait"=TRUE) -> ()  [unwired: 1 in, 5 out]
          }
        }
        n67 = local read "Start Scan"() -> (w83:bool)
        n68 = local read "Outphase Array"() -> (w100:dbl[][])
        n69 = local read "Inphase Array"() -> (w102:dbl[][])
        n70 = local read "Ratio Array"() -> (w104:dbl[][])
        n71 = Increment(x=w85) -> (x+1=w92:i32)
        n72 = Insert Into Array(array=w102, index (row)=w85, new element=w101) -> (w81:dbl[][])  [unwired: 1 in]
        "AI2" <- w81
        n73 = Insert Into Array(array=w100, index (row)=w85, new element=w84) -> (w99:dbl[][])  [unwired: 1 in]
        n74 = Insert Into Array(array=w104, index (row)=w85, new element=w103) -> (w82:dbl[][])  [unwired: 1 in]
        n75 = local write "Outphase Array"(w99) -> ()
        n76 = local write "Inphase Array"(w81) -> ()
        n77 = local write "Ratio Array"(w82) -> ()
        n78 = local read "Pixels(Y)"() -> (w97:i32)
        n79 = Less?(x=w92, y=w97) -> (x < y?=w91:bool)
        n80 = And(x=w83, y=w91) -> (x .and. y?=w90:bool)
        "x .and. y?" <- w90
        n81 = local read "Pixels(X)"() -> (w96:i32)
        n82 = property on="AI2" class="IntGraph (strict)"("X Scale.Range:Minimum"=w89, "X Scale.Range:Maximum"=w96, "Y Scale.Range:Minimum"=w89, "Y Scale.Range:Maximum"=w97, "Z Scale.Range:Minimum"="Z Scale.Range:Minimum", "Z Scale.Range:Maximum"="Z Scale.Range:Maximum") -> ()  [unwired: 2 in, 2 out]
      }
      n83 = disable-structure shown="Enabled" {
        disable-tunnel: w57 -> [w65 _]
        disable-tunnel: w56 -> [w64 _]
        disable-tunnel: w55 -> [w63 _]
        frame Enabled {
          n84 = stacked-sequence {
            tunnel: w65 -> [_ w75]
            tunnel: w64 -> [_ _]
            tunnel: w63 -> [_ _]
            frame #0 {
              n85 = call <vilib>:"Beep.vi"("use system alert? (T)"=FALSE, "duration (msec)"=300, "frequency (Hz)"=2093) -> ()  [unwired: 9 out]
              n86 = call <vilib>:"Beep.vi"("use system alert? (T)"=FALSE, "duration (msec)"=300, "frequency (Hz)"=3000) -> ()  [unwired: 9 out]
              n87 = call <vilib>:"Beep.vi"("use system alert? (T)"=FALSE, "duration (msec)"=300, "frequency (Hz)"=4186) -> ()  [unwired: 9 out]
            }
            frame #1 {
              # "AI2"
              n88 = Array Size(array=w75) -> (size(s)=w77:i32[])
              n89 = Multiply Array Elements(1:w77) -> (0:w76:i32)
              n90 = Reshape Array(w75, w76) -> (w78:dbl[])
              n91 = call-poly <vilib>:"Write Delimited Spreadsheet.vi"("file path (dialog if empty)"="Path", "format (%.3f)"="%.7f", "1D data"=w78) -> ()  [unwired: 11 in, 2 out]
            }
          }
        }
        frame Disabled {
        }
      }
    }
    frame #3 {
      # "Stop the Controls"
      n92 = local read "MG17Motor B"() -> (w178:refnum<k7>)
      n93 = local read "MG17Motor A"() -> (w180:refnum<k7>)
      n94 = invoke class="MG17Motor" method="StopCtrl"(reference=w180) -> (error out=w179:errorcluster)  [unwired: 2 in, 2 out]
      n95 = invoke class="MG17Motor" method="StopCtrl"(reference=w178, error in=w179) -> (error out=w181:errorcluster)  [unwired: 1 in, 2 out]
      n96 = local write "error"(w181) -> ()
    }
  }
  n97 = stacked-sequence {
    tunnel: [5120 ("buffer size (1000 scans)")] -> w1
    frame #0 {
    }
  }
  n98 = call-poly <vilib>:"DAQmx Create Virtual Channel.vi"("physical channels"="Physical Channel") -> ("task out"=w10:refnum<k21>, "error out"=w9:errorcluster)  [unwired: 8 in, 5 out]
  n99 = local write "x .and. y?"(TRUE) -> ()
  n100 = call-poly <vilib>:"DAQmx Timing.vi"("task/channels in"=w10, "sample mode"=w2, "samples per channel"=w1, "rate"="AI Rate", "error in"=w9) -> ("task out"=w8:refnum<k21>, "error out"=w7:errorcluster)  [unwired: 2 in, 7 out]
  n101 = Multiply(x="AI Rate", y=0.05) -> (x*y=w5:dbl)
  n102 = To Long Integer(number=w5) -> (32bit integer=w4:i32)
  n103 = call <vilib>:"DAQmx Start Task.vi"("task/channels in"=w8, "error in"=w7) -> ("task out"=w15:refnum<k21>, "error out"=w12:errorcluster)  [unwired: 12 out]
  n104 = while {
    tunnel: w15 -> [w201]
    tunnel: [w200] -> w13
    shift-right: [w198] -> w11
    shift-left: w12 -> [w198]
    tunnel: "AI Rate" -> [_]
    tunnel: w4 -> [w186]
    tunnel: "AI Rate" -> [_]
    stop <- FALSE stop-if-true
    n105 = call-poly <vilib>:"DAQmx Read.vi"("task/channels in"=w201, "number of samples per channel"=w186) -> ("task out"=w200:refnum<k21>, "data"=w190:dbl[][])  [unwired: 1 in, 11 out]
    "scaled data" <- w190
    n106 = Index Array(array=w190, index (row)=0 ("disabled index (col)")) -> (element=w184:dbl[])  [unwired: 1 in]
    n107 = Index Array(array=w190, index (row)=1) -> (element=w192:dbl[])  [unwired: 1 in]
    n108 = Index Array(array=w190, index (row)=2) -> (element=w187:dbl[])  [unwired: 1 in]
    n109 = Add Array Elements(numeric array=w187) -> (sum=w188:dbl)
    n110 = Add Array Elements(numeric array=w192) -> (sum=w193:dbl)
    n111 = Add Array Elements(numeric array=w184) -> (sum=w196:dbl)
    n112 = Array Size(array=w184) -> (size(s)=→"array size":i32)
    n113 = Divide(x=w188, y=w186) -> (x/y=→"AI2":dbl)
    n114 = Divide(x=w193, y=w186) -> (x/y=→"AI1":dbl)
    n115 = Divide(x=w196, y=w186) -> (x/y=→"AI0":dbl)
  }
  n116 = call <vilib>:"DAQmx Clear Task.vi"("task in"=w13, "error in"=w11) -> ("error out"=w14:errorcluster)  [unwired: 13 out]
  n117 = call <vilib>:"Simple Error Handler.vi"("error in (no error)"=w14) -> ()  [unwired: 1 in, 8 out]
